vi "Get Trigger Sense Div.vi"() -> (3 "function return":dbl)   [LabVIEW 2021, in "vmmso.lvlib"]
doc: "DLL_API double WINAPI GetTriggerSenseDiv();"
uses:
  vmmso.lvlib
  vmmso.dll
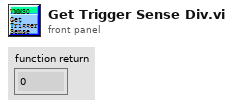
[diagram p1: front panel]
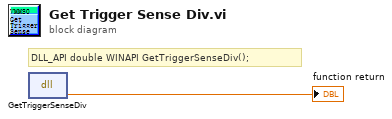
[diagram p0: block diagram]
diagram:
  # "DLL_API double WINAPI GetTriggerSenseDiv();"
  n1 = dll-call lib="D:/labviewdemo/LabviewDemo 21/vmmso/vmmso.*" fn="GetTriggerSenseDiv"() -> (→"function return":dbl)  [unwired: 3 in, 2 out]
